vi "Stop User Event LV2.vi"(0 "Stop":bool=TRUE, 11 "Error In":errorcluster, 13 "Operations":T1) -> (4 "Stop Out":refnum<user-event>, 15 "Error Out":errorcluster)   [LabVIEW 2021, in "Calculator.lvlib"]
doc: "This VI acts as an user event LV2 for handling with stop events."
uses:
  Calculator.lvlib
  Controls/User Event Operations.ctl
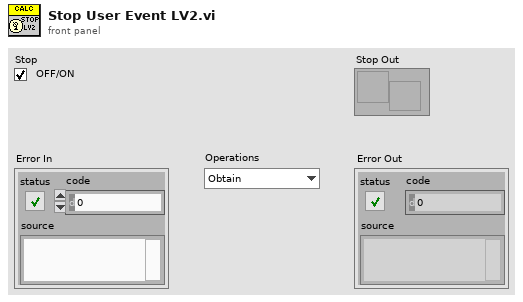
[diagram p1: front panel]
types:
  T1 = typedef "Calculator.lvlib/User Event Operations.ctl" = enum16{"Obtain", "Generate", "Release"}
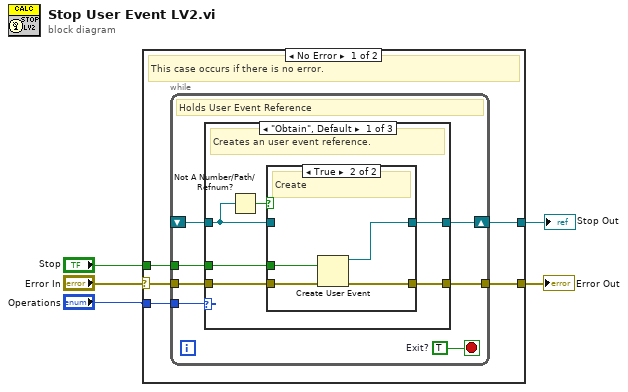
[diagram p0: block diagram]
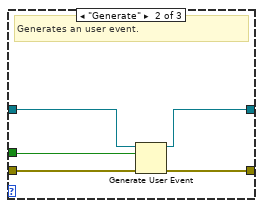
[diagram p3: hidden frame]
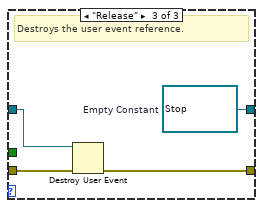
[diagram p4: hidden frame]
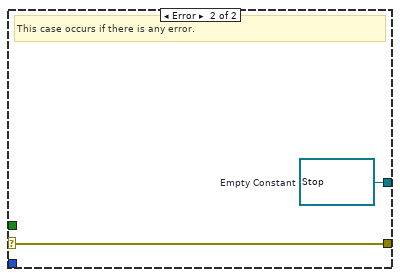
[diagram p5: hidden frame]
diagram:
  n1 = case shown="No Error" "Error In" {
    selector: "Error In" -> [w8 w40]
    tunnel: "Operations" -> [w10 _]
    tunnel: "Stop" -> [w9 _]
    tunnel: [w7 w40] -> w4
    tunnel: [w6 w39] -> w2
    frame No Error {
      # "This case occurs if there is no error."
      n2 = while {
        tunnel: w10 -> [w17]
        tunnel: w9 -> [w16]
        tunnel: w8 -> [w15]
        tunnel: [w14] -> w7
        shift-right: [w13] -> w6
        shift-left: _ -> [w12]
        stop <- w11 stop-if-true
        w11 = TRUE  # Exit?
        # "Holds User Event Reference"
        n3 = case shown="\"Obtain\", Default" w17 {
          tunnel: w16 -> [w21 w34 _]
          tunnel: w15 -> [w22 w33 w37]
          tunnel: [w23 w32 w38] -> w14
          tunnel: [w20 w30 w35] -> w13
          tunnel: w12 -> [w19 w31 w36]
          frame "Obtain", Default {
            # "Creates an user event reference."
            n4 = Not A Number/Path/Refnum?(number/path/refnum=w19) -> (NaN/Path/Refnum?=w18:bool)
            n5 = case shown="True" w18 {
              tunnel: [w24 w29] -> w23
              tunnel: w22 -> [w24 w28]
              tunnel: w21 -> [_ w27]
              tunnel: [w25 w26] -> w20
              tunnel: w19 -> [w25 _]
              frame False {
                # "Use existing"
              }
              frame True {
                # "Create"
                n6 = Create User Event(user event datatype=w27, error in=w28) -> (user event=w26:refnum<user-event>, error out=w29:errorcluster)
              }
            }
          }
          frame "Generate" {
            # "Generates an user event."
            n7 = Generate User Event(user event=w31, event data cluster=w34, error in=w33) -> (user event out=w30:refnum<user-event>, error out=w32:errorcluster)  [unwired: 1 in]
          }
          frame "Release" {
            w35 = refnum<user-event> refnum  # Empty Constant
            # "Destroys the user event reference."
            n8 = Destroy User Event(user event=w36, error in=w37) -> (error out=w38:errorcluster)
          }
        }
      }
    }
    frame Error {
      w39 = refnum<user-event> refnum  # Empty Constant
      # "This case occurs if there is any error."
    }
  }
  "Error Out" <- w4
  "Stop Out" <- w2
